vi "CLD 11 CSV file utility.vi"(8 "Error In":errorcluster, 10 "[Data In]":T1[](array[typedef]), 11 "CSV File Enum":T2) -> (0 "Error Out":errorcluster, 3 "[Data Out]":T1[](array[typedef]))   [LabVIEW 2009]
doc: "CLD 11 File utility from CLD 6"
uses:
  CLD 11 CSV file enum.ctl
  CLD 11 CSV file data structure.ctl
  <vilib>/Utility/file.llb/Read From Spreadsheet File (string).vi
  <vilib>/Utility/file.llb/Write To Spreadsheet File (string).vi
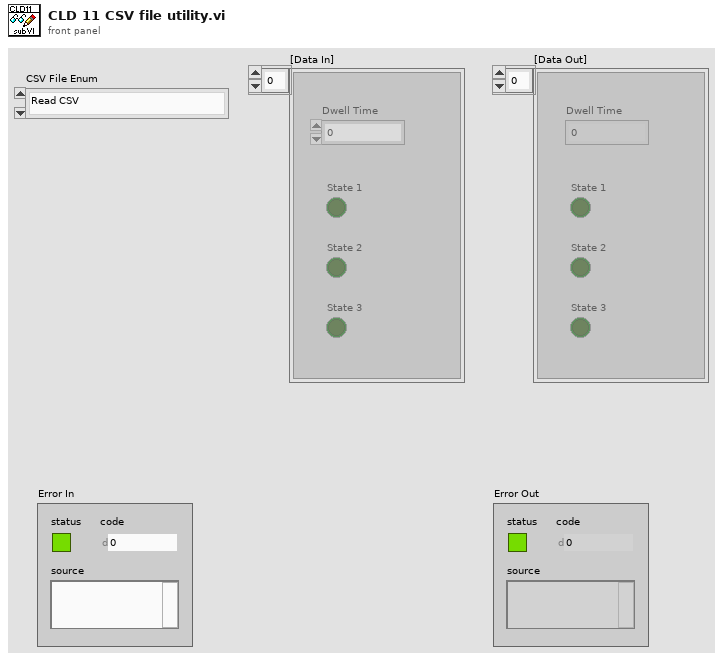
[diagram p1: front panel]
types:
  T1 = typedef "CLD 11 CSV file data structure.ctl" = cluster{"Dwell Time":i32, "State 1":bool, "State 2":bool, "State 3":bool}
  T2 = typedef "CLD 11 CSV file enum.ctl" = enum16{"Read CSV", "Write CSV"}
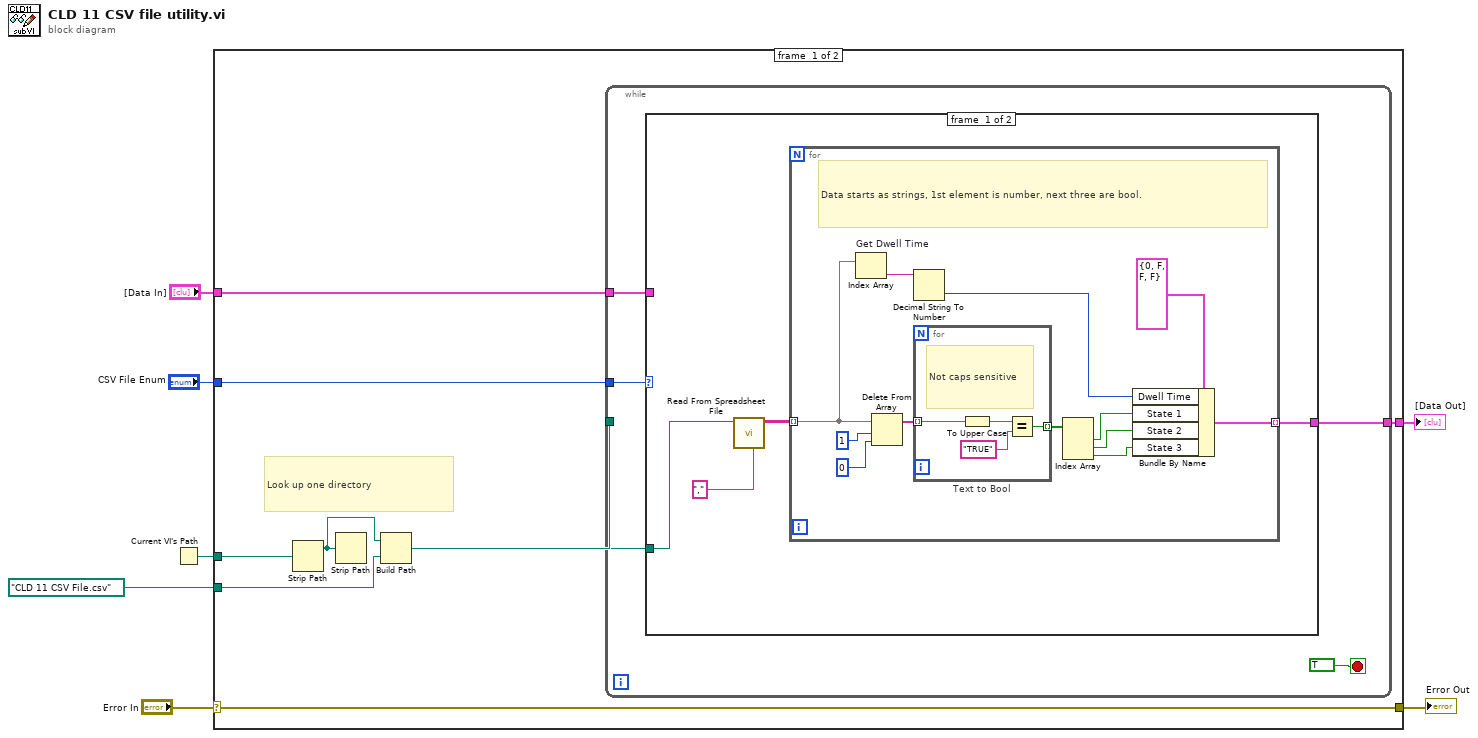
[diagram p0: block diagram]
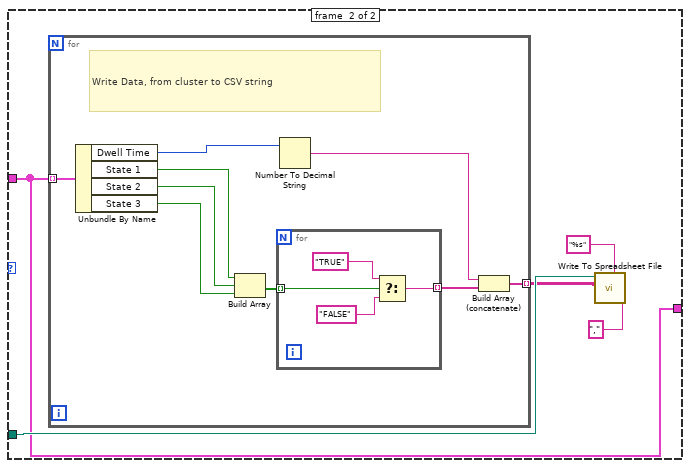
[diagram p2: hidden frame]
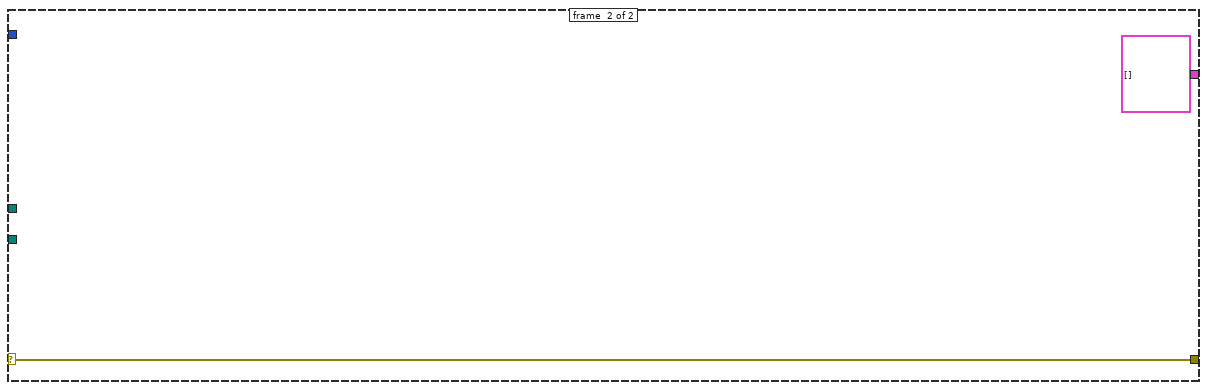
[diagram p3: hidden frame]
diagram:
  n1 = Current VI's Path() -> (path=w5:path)
  n2 = case shown="No Error" "Error In" {
    selector: "Error In" -> [w9 w60]
    tunnel: [w15 T1[] [] ("[Data In]")] -> w7
    tunnel: path "CLD 11 CSV File.csv" -> [w14 _]
    tunnel: w5 -> [w13 _]
    tunnel: "CSV File Enum" -> [w11 _]
    tunnel: "[Data In]" -> [w10 _]
    tunnel: [w9 w60] -> w1
    frame #0 {
      # "Look up one directory"
      n3 = Strip Path(path=w13) -> (stripped path=w8:path)  [unwired: 1 out]
      n4 = Strip Path(path=w8) -> ()  [unwired: 2 out]
      n5 = Build Path(base path=w8, name or relative path=w14) -> (appended path=w12:path)
      n6 = while {
        tunnel: w12 -> [w18]
        tunnel: w11 -> [w19]
        tunnel: [w17] -> w15
        tunnel: w10 -> [w16]
        stop <- TRUE stop-if-true
        n7 = case shown="\"Read CSV\", Default" w19 {
          tunnel: w18 -> [w24 w45]
          tunnel: [w22 w41] -> w17
          tunnel: w16 -> [_ w41]
          frame #0 {
            n8 = call-poly <vilib>:"Read From Spreadsheet File.vi"("delimiter (\\t)"="," ("delimiter (\\t)"), "file path (dialog if empty)"=w24) -> ("all rows"=w23:string[][])  [unwired: 5 in, 4 out]
            n9 = for {
              tunnel: w23 -> [w33] mode=indexing
              tunnel: [w36] -> w22 mode=indexing
              # "Data starts as strings, 1st element is number, next three are bool."
              n10 = Index Array "Get Dwell Time"(array=w33) -> (element=w35:string)  [unwired: 1 in]
              n11 = Delete From Array(array=w33, length=1, index=0) -> (array with subset deleted=w26:string[])  [unwired: 1 out]
              n12 = Decimal String To Number(string=w35) -> (number=w34:i32)  [unwired: 2 in, 1 out]
              n13 = for "Text to Bool" {
                tunnel: w26 -> [w40] mode=indexing
                tunnel: [w37] -> w30 mode=indexing
                # "Not caps sensitive"
                n14 = To Upper Case(1:w40) -> (0:w39:string)
                n15 = Equal?(x=w39, y="TRUE") -> (x = y?=w37:bool)
              }
              n16 = Index Array(array=w30) -> (element #1=w29:bool, element #2=w28:bool, element #3=w27:bool)  [unwired: 3 in]
              n17 = Bundle By Name(cluster=T1 {"Dwell Time"=0, "State 1"=FALSE, "State 2"=FALSE, "State 3"=FALSE} ("CSV File Data Structure"), "Dwell Time"=w34, "State 1"=w29, "State 2"=w28, "State 3"=w27) -> (w36:T1)
            }
          }
          frame #1 {
            n18 = for {
              tunnel: w41 -> [w54] mode=indexing
              tunnel: [w46] -> w43 mode=indexing
              # "Write Data, from cluster to CSV string"
              n19 = Unbundle By Name(w54) -> ("Dwell Time"=w53:i32, "State 1"=w52:bool, "State 2"=w51:bool, "State 3"=w50:bool)
              n20 = Build Array(w52, w51, w50) -> (w49:bool[])
              n21 = for {
                tunnel: w49 -> [w58] mode=indexing
                tunnel: [w55] -> w47 mode=indexing
                n22 = Select(t="TRUE", s=w58, f="FALSE") -> (s? t:f=w55:string)
              }
              n23 = Number To Decimal String(number=w53) -> (decimal integer string=w48:string)  [unwired: 1 in]
              n24 = Build Array (concatenate)(w48, w47) -> (w46:string[])
            }
            n25 = call-poly <vilib>:"Write To Spreadsheet File.vi"("delimiter (\\t)"="," ("delimiter (\\t)"), "format (%s)"="%s", "2D data"=w43, "file path (dialog if empty)"=w45) -> ()  [unwired: 4 in, 1 out]
          }
        }
      }
    }
    frame #1 {
    }
  }
  "[Data Out]" <- w7
  "Error Out" <- w1
